vi "AlliGator Set Loaded Image Resolution.vi"(7 "Image Characteristics in (Default)":T1={"Calibration"={"X Step"=0.0, "Y Step"=0.0, "Unit"=enum."Undefined"}, "File Type"="TIFF", "X Resolution"=0, "Y Resolution"=0, "File Data Type"=5, "Image Type"=2} {"Calibration"."Y Step" format="%.2f"; "Calibration"."X Step" format="%.2f"; "Image Type" items=["Grayscale (U8)", "Grayscale (I16)", "Grayscale (SGL)", "Complex (CSG)", "RGB (U32)", "HSL (U32)", "RGB (U64)", "Grayscale (U16)"]}, 8 "Error In":errorcluster, 9 "Image Y":i32, 10 "Image X":i32, 11 "Image Loading Options":T5 {"Hot Pixel Removal"."Percentile" min=0 max=100; "Image Binning Options"."Y Bin" min=1; "Image Binning Options"."X Bin" min=1; "Image Smoothing Options"."Bin" min=1}) -> (0 "Error Out":errorcluster, 3 "Image Characteristics":T1 {"Calibration"."Y Step" format="%.2f"; "Calibration"."X Step" format="%.2f"; "Image Type" items=["Grayscale (U8)", "Grayscale (I16)", "Grayscale (SGL)", "Complex (CSG)", "RGB (U32)", "HSL (U32)", "RGB (U64)", "Grayscale (U16)"]})   [LabVIEW 2021, in "AlliGator Source Image.lvlib"]
doc: "Sets the loaded image's resolution from the provided information."
uses:
  AlliGator Source Image.lvlib
  AlliGator Image Loading Options.ctl
  Settings/AlliGator Image Smoothing Options.ctl
  Arrays/Kernel Type.ctl
  Arrays/Smoothing Algorithm.ctl
  Settings/AlliGator Background Subtraction Parameters.ctl
  AlliGator Image Binning Options.ctl
  Settings/AlliGator Gates to Keep.ctl
  SwissSPAD/SwissSPAD Live_Image Display Options.ctl
  Files/AlliGator Image Pre-processing Step.ctl
  Image/Image Characteristics.ctl
  Arrays/Arrays.lvlib
  Settings/AlliGator Settings.lvlib
  Image/Image.lvlib
  SwissSPAD/SwissSPAD Live.lvlib
  Files/AlliGator Files.lvlib
panel:
  # "Image Type >> Grayscale (SGL)"
  # "see the AlliGator License on the block diagram (Ctrl+E or Window:Show Block Diagram)"
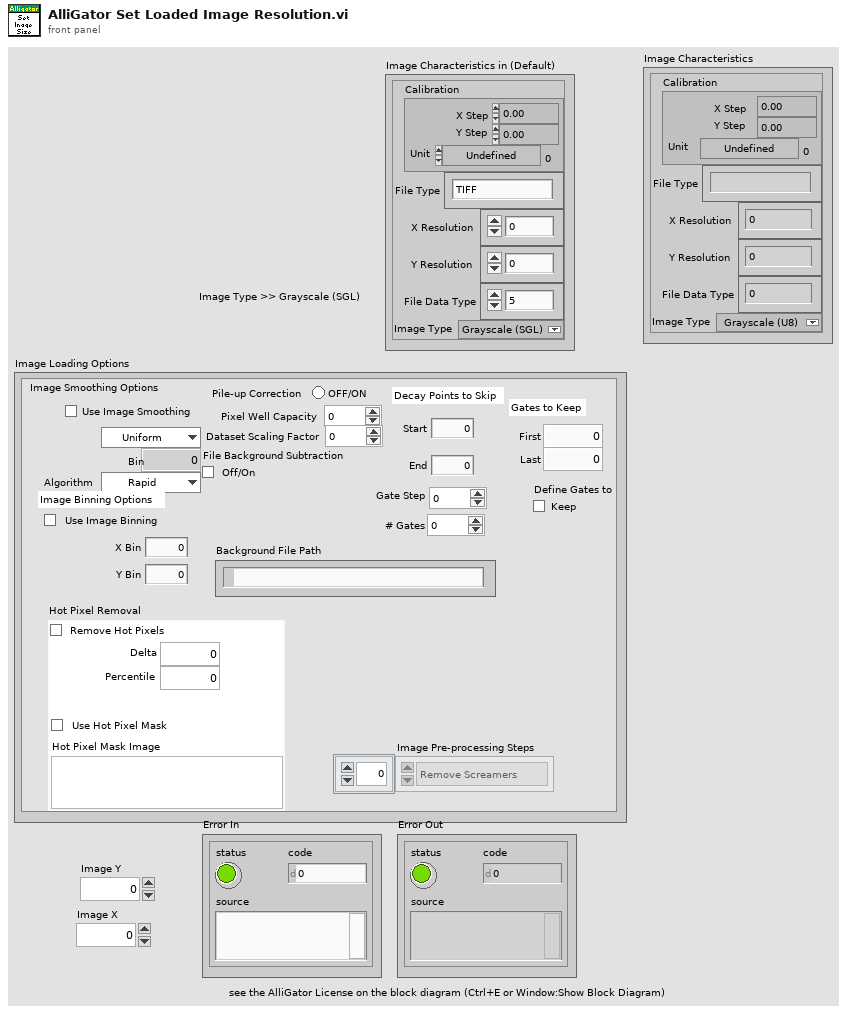
[diagram p1: front panel]
types:
  T1 = typedef "Image.lvlib/Image Characteristics.ctl" = cluster{"Calibration":T2, "File Type":string, "X Resolution":i32, "Y Resolution":i32, "File Data Type":i32, "Image Type":T4}
  T2 = typedef "Simple Grid Descriptor" = cluster{"X Step":sgl, "Y Step":sgl, "Unit":T3}
  T3 = typedef "Image Unit" = enum32{"Undefined", "Angström", "Micrometer", "Millimeter", "Centimeter", "Meter", "Kilometer", "Microinch", "Inch", "Feet", "Nautical miles", "Standard miles", "Steps"}
  T4 = typedef "Image Type" = u32
  T5 = typedef "AlliGator Source Image.lvlib/AlliGator Image Loading Options.ctl" = cluster{"Pixel Well Capacity":u32, "Pile-up Correction":bool, "Gate Step":i32, "Image Smoothing Options":T6, "Gates to Skip":T9, "File Background Subtraction":bool, "Background File Path":path, "Image Binning Options":T10, "# Gates":u32, "Gates to Keep":T11, "Define Gates to":bool, "Hot Pixel Removal":T12, "Dataset Scaling Factor":dbl, "Image Pre-processing Steps":T13[]}
  T6 = typedef "AlliGator Settings.lvlib/AlliGator Image Smoothing Options.ctl" = cluster{"Use Image Smoothing":bool, "Kernel Type":T7, "Bin":i32, "Algorithm":T8}
  T7 = typedef "Arrays.lvlib/Kernel Type.ctl" = enum16{"Uniform", "Bilinear", "Gaussian"}
  T8 = typedef "Arrays.lvlib/Smoothing Algorithm.ctl" = enum16{"Rapid", "Thorough"}
  T9 = typedef "AlliGator Settings.lvlib/AlliGator Background Subtraction Parameters.ctl" = cluster{"Start":u32, "End":u32}
  T10 = typedef "AlliGator Source Image.lvlib/AlliGator Image Binning Options.ctl" = cluster{"Use Image Binning":bool, "X Bin":i32, "Y Bin":i32}
  T11 = typedef "AlliGator Settings.lvlib/AlliGator Gates to Keep.ctl" = cluster{"First":u32, "Last":u32}
  T12 = typedef "SwissSPAD Live.lvlib/SwissSPAD Live_Image Display Options.ctl" = cluster{"Remove Screamers":bool, "Delta":sgl, "Equalize Histogram":bool, "Percentile":sgl, "Hot Pixel Mask Image":path, "Use Hot Pixel Mask":bool}
  T13 = typedef "AlliGator Files.lvlib/AlliGator Image Pre-processing Step.ctl" = enum16{"Remove Screamers", "Pile-up Correction", "Binning", "Smoothing", "Rescaling", "Dead Left Column Correction"}
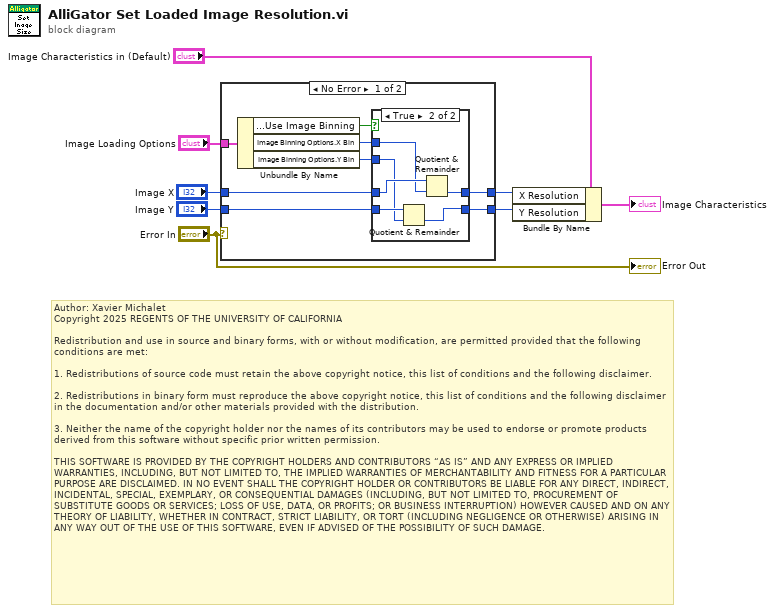
[diagram p0: block diagram]
diagram:
  # "Author: Xavier Michalet\nCopyright 2025 REGENTS OF THE UNIVERSITY OF CALIFORNIA\n\nRedistribution and use in source and binary forms, with or without modification, are permitted provided that the following conditions are met:\n\n1. Redistributions of source code must retain the above copyright notice, this list of conditions and the following disclaimer.\n\n2. Redistributions in binary form must reproduce the above copyright notice, this list of conditions and the following disclaimer in the documentation and/or other materials provided with the distribution.\n\n3. Neither the name of the copyright holder nor the names of its contributors may be used to endorse or promote products derived from this software without specific prior written permission.\n\nTHIS SOFTWARE IS PROVIDED BY THE COPYRIGHT HOLDERS AND CONTRIBUTORS “AS IS” AND ANY EXPRESS OR IMPLIED WARRANTIES, INCLUDING, BUT NOT LIMITED TO, THE IMPLIED WARRANTIES OF MERCHANTABILITY AND FITNESS FOR A PARTICULAR PURPOSE ARE DISCLAIMED. IN NO EVENT SHALL THE COPYRIGHT HOLDER OR CONTRIBUTORS BE LIABLE FOR ANY DIRECT, INDIRECT, INCIDENTAL, SPECIAL, EXEMPLARY, OR CONSEQUENTIAL DAMAGES (INCLUDING, BUT NOT LIMITED TO, PROCUREMENT OF SUBSTITUTE GOODS OR SERVICES; LOSS OF USE, DATA, OR PROFITS; OR BUSINESS INTERRUPTION) HOWEVER CAUSED AND ON ANY THEORY OF LIABILITY, WHETHER IN CONTRACT, STRICT LIABILITY, OR TORT (INCLUDING NEGLIGENCE OR OTHERWISE) ARISING IN ANY WAY OUT OF THE USE OF THIS SOFTWARE, EVEN IF ADVISED OF THE POSSIBILITY OF SUCH DAMAGE."
  n1 = case shown="No Error" "Error In" {
    tunnel: "Image Loading Options" -> [w16 _]
    tunnel: "Image X" -> [w12 w26]
    tunnel: "Image Y" -> [w11 w25]
    tunnel: [w10 w26] -> w3
    tunnel: [w9 w25] -> w2
    frame No Error {
      n2 = Unbundle By Name(w16) -> ("Image Binning Options.Use Image Binning"=w15:bool, "Image Binning Options.X Bin"=w14:i32, "Image Binning Options.Y Bin"=w13:i32)
      n3 = case shown="True" w15 {
        tunnel: w14 -> [_ w23]
        tunnel: w13 -> [_ w21]
        tunnel: w12 -> [w18 w24]
        tunnel: w11 -> [w17 w22]
        tunnel: [w18 w19] -> w10
        tunnel: [w17 w20] -> w9
        frame False {
        }
        frame True {
          n4 = Quotient & Remainder(x=w22, y=w21) -> (floor(x/y)=w20:i32)  [unwired: 1 out]
          n5 = Quotient & Remainder(x=w24, y=w23) -> (floor(x/y)=w19:i32)  [unwired: 1 out]
        }
      }
    }
    frame Error {
    }
  }
  n6 = Bundle By Name(cluster="Image Characteristics in (Default)", "X Resolution"=w3, "Y Resolution"=w2) -> (→"Image Characteristics":T1)
  "Error Out" <- "Error In"
